vi "Write Test Stand Class.vi"(8 "error in (no error)":errorcluster, 10 "Generic Test Stand":refnum<class "Generic Test Stand.lvclass">, 11 "Init DAC Process in":refnum<class "Init DAC Process.lvclass">) -> (0 "error out":errorcluster, 3 "Init DAC Process out":refnum<class "Init DAC Process.lvclass">)   [LabVIEW 2019, in "DAC Process.lvlib" / "Init DAC Process.lvclass"]
uses:
  Init DAC Process.lvclass
  Generic Test Stand/Generic Test Stand.lvclass
  Init DAC Process.lvclass/Init DAC Process.ctl
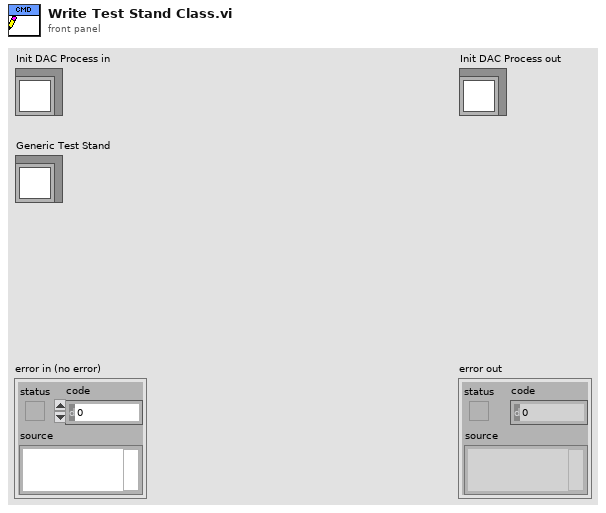
[diagram p1: front panel]
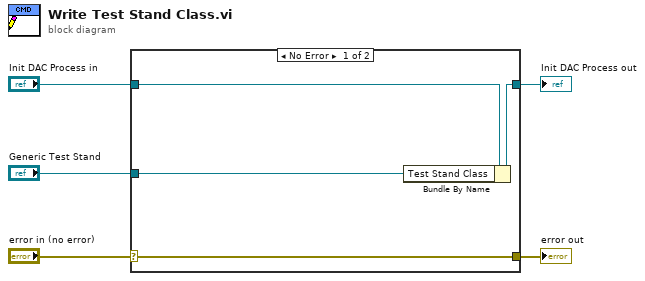
[diagram p0: block diagram]
diagram:
  n1 = case shown="No Error" "error in (no error)" {
    selector: "error in (no error)" -> [w9 w10]
    tunnel: [w9 w10] -> w4
    tunnel: [w7 w11] -> w2
    tunnel: "Init DAC Process in" -> [w8 w11]
    tunnel: "Generic Test Stand" -> [w6 _]
    frame No Error {
      n2 = Bundle By Name(cluster=w8, "Test Stand Class"=w6) -> (w7:refnum<class "Init DAC Process.lvclass">)
    }
    frame Error {
    }
  }
  "error out" <- w4
  "Init DAC Process out" <- w2
